vi "Setup Statically-Linked subWorkers.vi"(8 "error in":errorcluster, 11 "Debug Server in":refnum<class "Debug Server.lvclass">) -> (0 "error out":errorcluster, 3 "Debug Server out":refnum<class "Debug Server.lvclass">)   [LabVIEW 2017, in "Debug Server.lvclass"]
doc: "<b>Note: Do not change the code in this VI!</b>\nThis VI performs a setup of all the statically-linked subWorkers that belong to the Worker that calls this VI. This VI is created automatically by the 'Create/Add Worker' tool and must be called <b>before</b> any statically linked subWorkers are called."
uses:
  Debug Server.lvclass
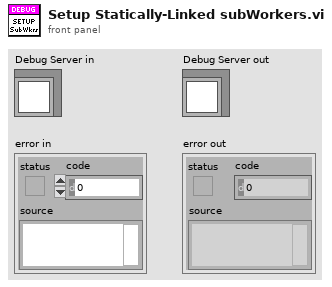
[diagram p1: front panel]
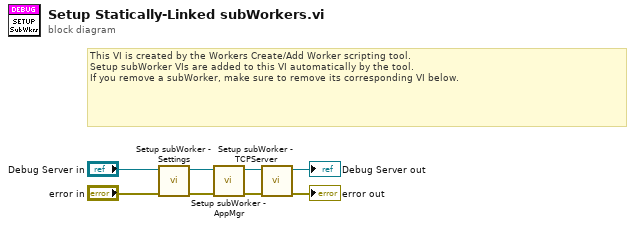
[diagram p0: block diagram]
diagram:
  # "This VI is created by the Workers Create/Add Worker scripting tool.\nSetup subWorker VIs are added to this VI automatically by the tool.\nIf you remove a subWorker, make sure to remove its corresponding VI below."
  n1 = call "Setup subWorker - Settings.vi"("error in"="error in", "Debug Server in"="Debug Server in") -> ("error out"=w7:errorcluster, "Debug Server out"=w4:refnum<class "Debug Server.lvclass">)  [unwired: 8 in]
  n2 = call "Setup subWorker - AppMgr.vi"("error in"=w7, "Debug Server in"=w4) -> ("error out"=w5:errorcluster, "Debug Server out"=w2:refnum<class "Debug Server.lvclass">)  [unwired: 8 in]
  n3 = call "Setup subWorker - TCPServer.vi"("error in"=w5, "Debug Server in"=w2) -> ("error out"=→"error out":errorcluster, "Debug Server out"=→"Debug Server out":refnum<class "Debug Server.lvclass">)  [unwired: 8 in]
